vi "Queue Driver.vi"(0 "State In":string, 5 "Data In":variant, 7 "EnqueueN States":string[](array[string]), 11 "error in (no error)":errorcluster, 13 "Queue Operation":T1) -> (4 "State Out":string, 6 "Data Out":variant, 15 "error out":errorcluster)   [LabVIEW 2019, in "Queue Driver.lvlib"]
uses:
  Queue Driver.lvlib
  Queue Operation.ctl
  Queue Data.ctl
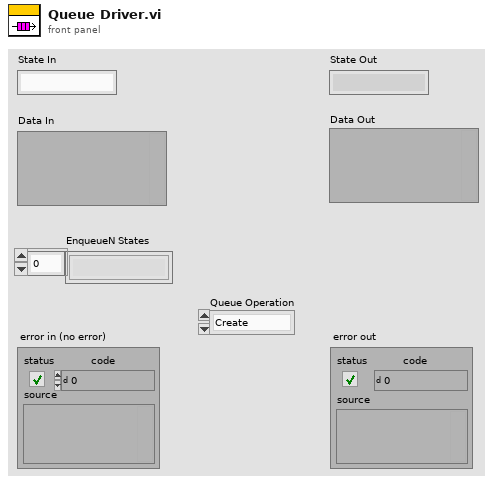
[diagram p1: front panel]
types:
  T1 = typedef "Queue Driver.lvlib/Queue Operation.ctl" = enum16{"Create", "Enqueue", "EnqueueN", "Dequeue", "Flush", "Destroy"}
  T2 = typedef "Queue Driver.lvlib/Queue Data.ctl" = cluster{"State":string, "Data":variant}
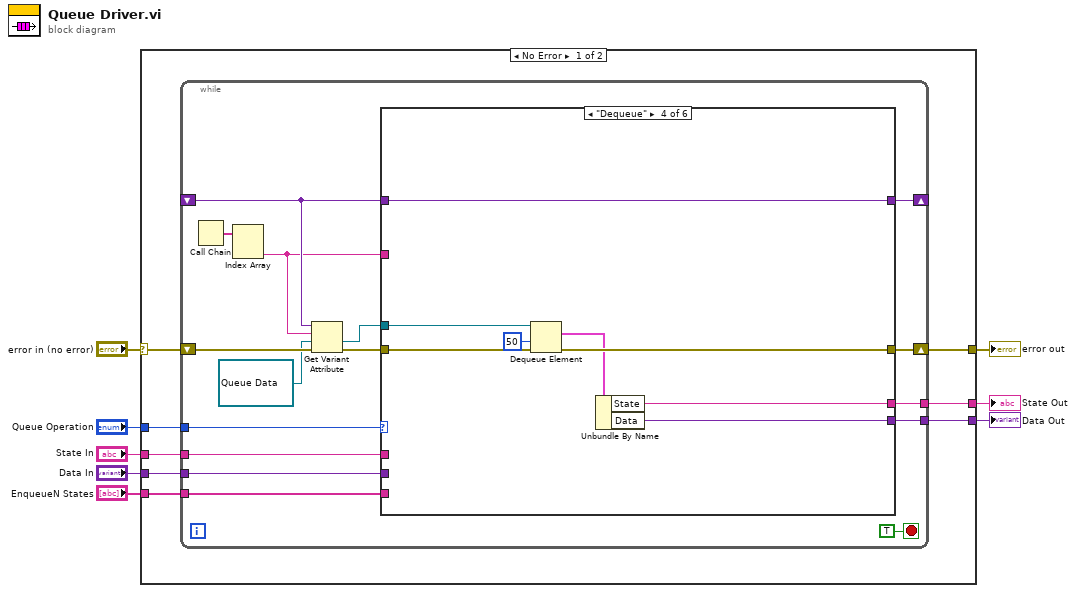
[diagram p0: block diagram]
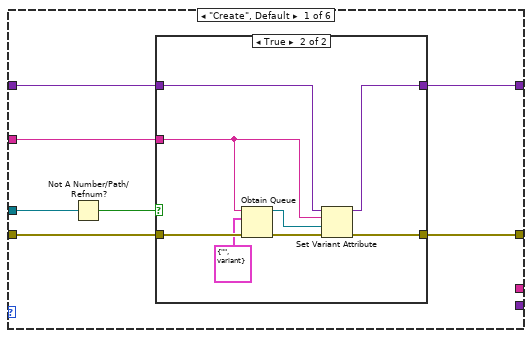
[diagram p2: hidden frame]
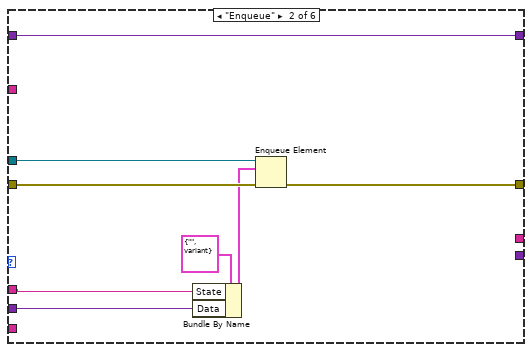
[diagram p4: hidden frame]
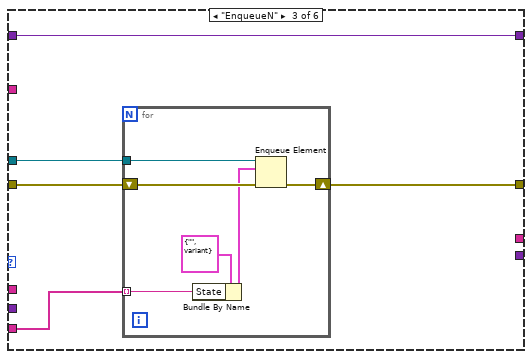
[diagram p5: hidden frame]
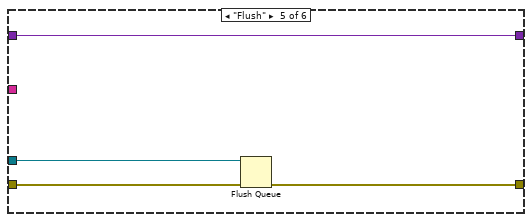
[diagram p6: hidden frame]
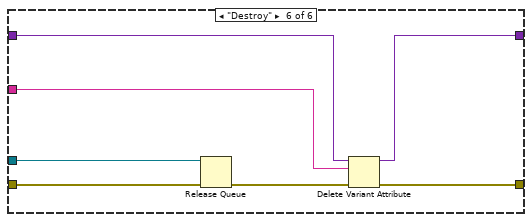
[diagram p7: hidden frame]
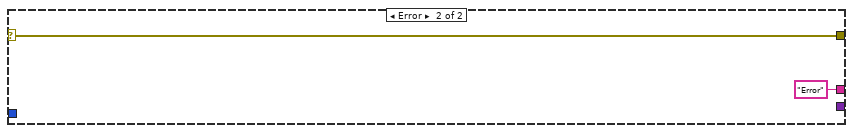
[diagram p8: hidden frame]
diagram:
  n1 = case shown="No Error" "error in (no error)" {
    selector: "error in (no error)" -> [w15 w89]
    tunnel: "Queue Operation" -> [w16 _]
    tunnel: "State In" -> [w14 _]
    tunnel: "Data In" -> [w13 _]
    tunnel: [w12 w89] -> w4
    tunnel: [w11 "Error" ("State")] -> w3
    tunnel: [w10 _] -> w2
    tunnel: "EnqueueN States" -> [w9 _]
    frame No Error {
      n2 = while {
        tunnel: w16 -> [w32]
        shift-right: [w23] -> _
        shift-left: _ -> [w28]
        shift-right: [w24] -> w12
        shift-left: w15 -> [w29]
        tunnel: w14 -> [w21]
        tunnel: w13 -> [w20]
        tunnel: [w19] -> w11
        tunnel: [w18] -> w10
        tunnel: w9 -> [w17]
        stop <- TRUE stop-if-true
        n3 = Call Chain() -> (call chain=w31:string[])
        n4 = Index Array(array=w31) -> (element #2=w25:string)  [unwired: 2 in, 1 out]
        n5 = Get Variant Attribute(Variant=w28, name=w25, default value (empty Variant)=refnum<queue> refnum ("queue out"), error in=w29) -> (value=w26:refnum<queue>, error out=w30:errorcluster)  [unwired: 2 out]
        n6 = case shown="\"Dequeue\"" w32 {
          tunnel: w30 -> [w39 w56 w61 w75 w78 w87]
          tunnel: w28 -> [w34 w57 w62 w76 w80 w82]
          tunnel: w26 -> [w38 w55 w60 w74 w77 w86]
          tunnel: w25 -> [w36 _ _ _ _ w81]
          tunnel: [w35 w50 w59 w73 w79 w84] -> w24
          tunnel: [w33 w57 w62 w76 w80 w83] -> w23
          tunnel: w21 -> [_ w53 _ _ _ _]
          tunnel: w20 -> [_ w52 _ _ _ _]
          tunnel: [_ _ _ w71 _ _] -> w19
          tunnel: [_ _ _ w70 _ _] -> w18
          tunnel: w17 -> [_ _ w58 _ _ _]
          frame "Create", Default {
            n7 = Not A Number/Path/Refnum?(number/path/refnum=w38) -> (NaN/Path/Refnum?=w37:bool)
            n8 = case shown="True" w37 {
              tunnel: w39 -> [w41 w49]
              tunnel: w36 -> [_ w43]
              tunnel: [w41 w46] -> w35
              tunnel: w34 -> [w40 w45]
              tunnel: [w40 w42] -> w33
              frame False {
              }
              frame True {
                n9 = Obtain Queue(name (unnamed)=w43, element data type=T2 {"State"="", "Data"=variant} ("Queue Data"), error in (no error)=w49) -> (queue out=w44:refnum<queue>, error out=w47:errorcluster)  [unwired: 2 in, 1 out]
                n10 = Set Variant Attribute(Variant=w45, name=w43, value=w44, error in=w47) -> (Variant out=w42:variant, error out=w46:errorcluster)  [unwired: 1 out]
              }
            }
          }
          frame "Enqueue" {
            n11 = Bundle By Name(cluster=T2 {"State"="", "Data"=variant} ("Queue Data"), "State"=w53, "Data"=w52) -> (w51:T2)
            n12 = Enqueue Element(queue=w55, element=w51, error in (no error)=w56) -> (error out=w50:errorcluster)  [unwired: 1 in, 2 out]
          }
          frame "EnqueueN" {
            n13 = for {
              tunnel: w60 -> [w67]
              shift-right: [w64] -> w59
              shift-left: w61 -> [w68]
              tunnel: w58 -> [w63] mode=indexing
              n14 = Bundle By Name(cluster=T2 {"State"="", "Data"=variant} ("Queue Data"), "State"=w63) -> (w65:T2)
              n15 = Enqueue Element(queue=w67, element=w65, error in (no error)=w68) -> (error out=w64:errorcluster)  [unwired: 1 in, 2 out]
            }
          }
          frame "Dequeue" {
            n16 = Dequeue Element(queue=w74, timeout in ms (-1)=50, error in (no error)=w75) -> (element=w72:T2, error out=w73:errorcluster)  [unwired: 2 out]
            n17 = Unbundle By Name(w72) -> ("State"=w71:string, "Data"=w70:variant)
          }
          frame "Flush" {
            n18 = Flush Queue(queue=w77, error in (no error)=w78) -> (error out=w79:errorcluster)  [unwired: 2 out]
          }
          frame "Destroy" {
            n19 = Release Queue(queue=w86, error in (no error)=w87) -> (error out=w85:errorcluster)  [unwired: 1 in, 2 out]
            n20 = Delete Variant Attribute(4:w85, 6:w81, 7:w82) -> (0:w84:errorcluster, 3:w83:variant)  [unwired: 1 out]
          }
        }
      }
    }
    frame Error {
    }
  }
  "error out" <- w4
  "State Out" <- w3
  "Data Out" <- w2
